vi "Image or Table Caption V2.vi"(0 "PDF Report IN":refnum<class "PDF Report Class.lvclass">, 2 "Image or Table":T1, 9 "Caption IN":string, 11 "error IN":errorcluster) -> (4 "PDF Report OUT":refnum<class "PDF Report Class.lvclass">, 6 "PdfpTable Refnum":refnum<k24>, 15 "error OUT":errorcluster)   [LabVIEW 2019, in "Exaprom PDF.lvlib"]
doc: "Version 2.0\nDeveloped by Jean-Marc Simard\nCopyright © 2012, Exaprom Inc.\nAll rights reserved.\nLicense: BSD\n\nWith iTextSharp 4.1.6 (http://itextsharp.sourceforge.net)\nunder Mozilla Public License Version 1.1\n(http://www.mozilla.org/MPL/MPL-1.1.html)"
uses:
  LV Class/PDF Report Class/PDF Report Class.lvclass
  C:/work/niobrara_lv/labview pdf writer fixing/DLL/itextsharp.dll
  DLL/itextsharp.dll
  Not  in the library/Images for controls/Image or Table.ctl
  Controls/Table Controls/Table properties.ctl
  Controls/Table Controls/Table position.ctl
  Controls/Table Controls/Cell, Alignment, LS and Font.ctl
  Controls/Table Controls/Cell Alignment 20px.ctl
  Controls/Table Controls/Text vertical arrangement.ctl
  Controls/Text Controls/Line spacing.ctl
  Controls/Table Controls/Merge Horizontal.ctl
  Controls/Font Controls/Font complete cluster.ctl
  Controls/Font Controls/Font size.ctl
  Controls/Font Controls/Font color.ctl
  Controls/Font Controls/Type and encoding.ctl
  Controls/Text Controls/Unicode/Type and run direction.ctl
  Controls/Table Controls/Cell Cluster.ctl
  Exaprom PDF.lvlib
  Controls/Table Controls/Cell Appearance.ctl
  Controls/Table Controls/Cell Border 20 px.ctl
  Controls/Table Controls/Cell Type, Alignment and LS.ctl
  Controls/Table Controls/Merge Vertical.ctl
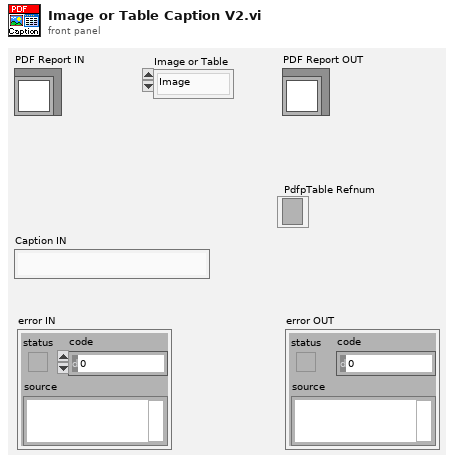
[diagram p1: front panel]
types:
  T1 = typedef "Exaprom PDF.lvlib/Image or Table.ctl" = enum16{"Image", "Table"}
  T2 = typedef "Exaprom PDF.lvlib/Cell Cluster.ctl" = cluster{"Font Ref":refnum<k24>, "Close font ref":bool, "Type and run direction":T3, "Cell Alignment":T4, "Text rotation":T5, "Leading":T6, "PdfP Cell ref":refnum<k24>, "Colspan":i8}
  T3 = typedef "Exaprom PDF.lvlib/Type and run direction.ctl" = enum16{"Select", "ASCII", "UTF-16", "UTF-16 (default)", "UTF-16 (LTR)", "UTF-16 (RTL)"}
  T4 = typedef "Exaprom PDF.lvlib/Cell Alignment 20px.ctl" = u16
  T5 = typedef "Exaprom PDF.lvlib/Text vertical arrangement.ctl" = enum16{"None", "Clockwise", "Counterclockwise"}
  T6 = typedef "Exaprom PDF.lvlib/Font size.ctl" = sgl
  T7 = cluster{"Row":cluster{"#":i16, "to #":i16}, "Cell [ ]":T2[]}
  T8 = typedef "Exaprom PDF.lvlib/Cell, Alignment, LS and Font.ctl" = cluster{"Text":T9, "Cell Appearance":T11, "HMerge":T13, "VMerge":T14, "Font":T15}
  T9 = typedef "Exaprom PDF.lvlib/Cell Type, Alignment and LS.ctl" = cluster{"Cell Alignment":T4, "Text rotation":T5, "Line spacing":T10}
  T10 = typedef "Exaprom PDF.lvlib/Line spacing.ctl" = enum16{"Select", "1.0", "1.5", "2.0"}
  T11 = typedef "Exaprom PDF.lvlib/Cell Appearance.ctl" = cluster{"Border":T12, "Thickness":sgl, "Color":u32, "BG":u32}
  T12 = typedef "Exaprom PDF.lvlib/Cell Border 20 px.ctl" = u16
  T13 = typedef "Exaprom PDF.lvlib/Merge Horizontal.ctl" = cluster{"From":i8, "to":i8}
  T14 = typedef "Exaprom PDF.lvlib/Merge Vertical.ctl" = cluster{"From":i8, "to":i8}
  T15 = typedef "Exaprom PDF.lvlib/Font complete cluster.ctl" = cluster{"Name":string, "Size":T6, "Color":T16, "Style":cluster{"Bold":bool, "Italic":bool, "Underline":bool, "Strikeout":bool}, "Type":T17}
  T16 = typedef "Exaprom PDF.lvlib/Font color.ctl" = u32
  T17 = typedef "Exaprom PDF.lvlib/Type and encoding.ctl" = cluster{"Type&direction":T3, "Embedded":bool, "Encoding":string}
  T18 = typedef "Exaprom PDF.lvlib/Table properties.ctl" = cluster{"Table position":T19, "SpacingBefore (points)":sgl, "SpacingAfter (points)":sgl}
  T19 = typedef "Exaprom PDF.lvlib/Table position.ctl" = i32
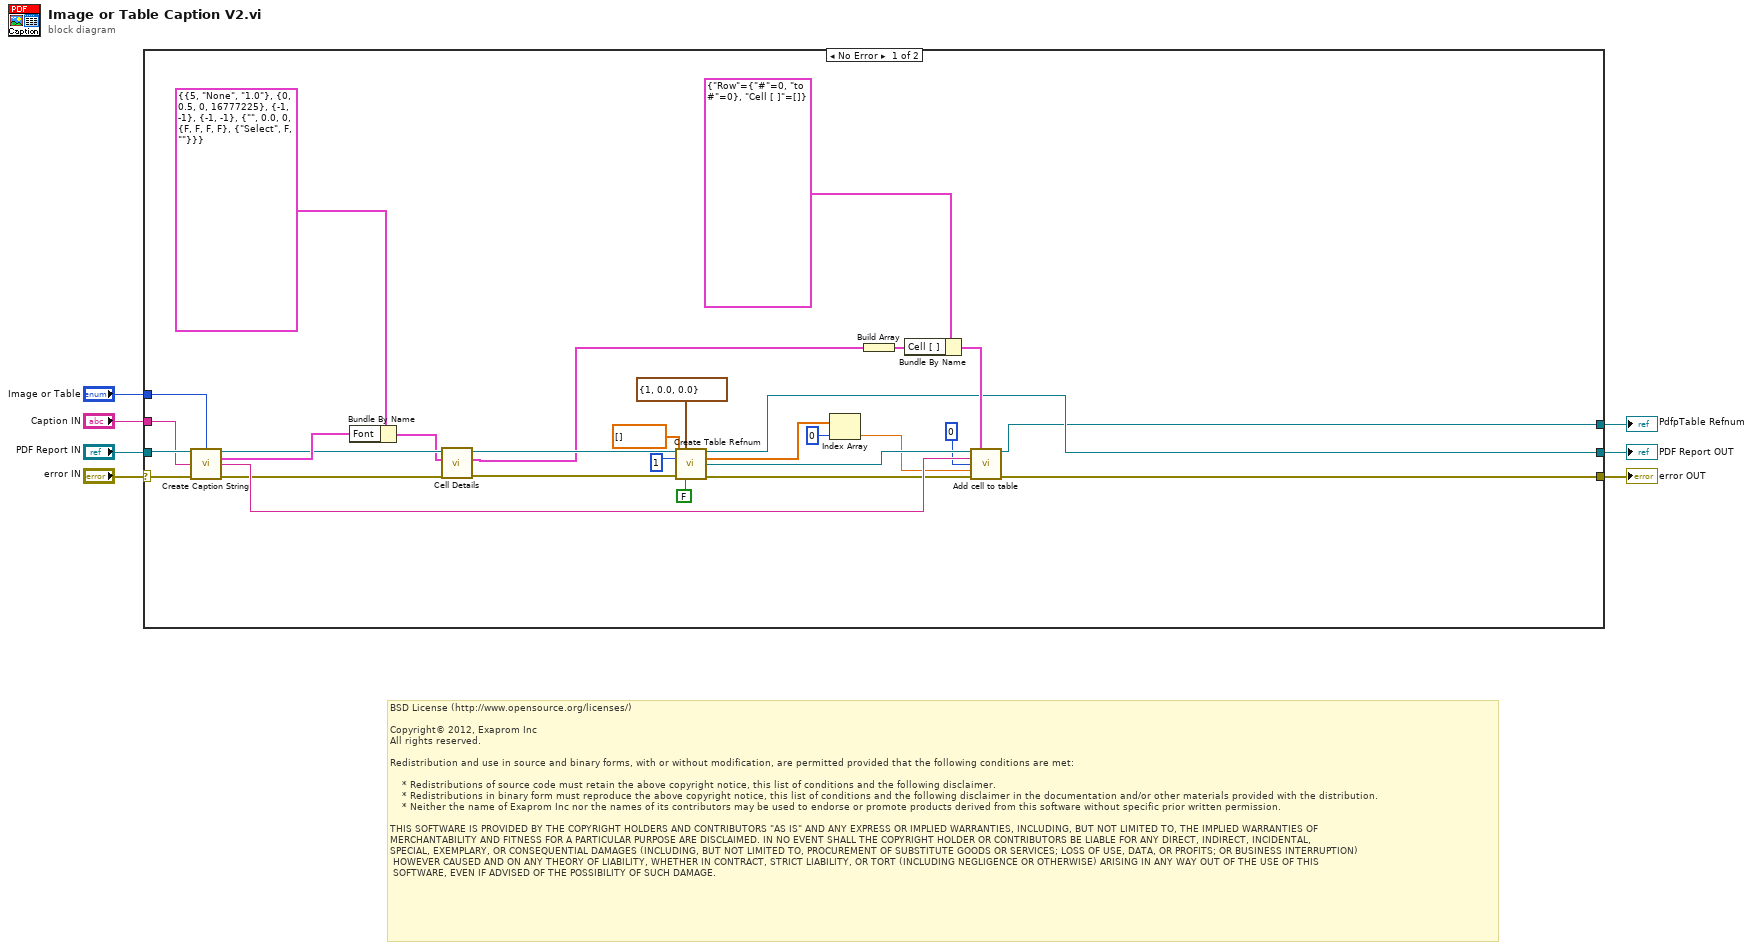
[diagram p0: block diagram]
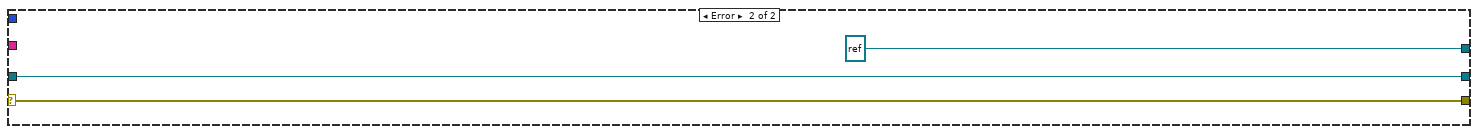
[diagram p2: hidden frame]
diagram:
  # "BSD License (http://www.opensource.org/licenses/)\n\nCopyright© 2012, Exaprom Inc\nAll rights reserved.\n\nRedistribution and use in source and binary forms, with or without modification, are permitted provided that the following conditions are met:\n\n    * Redistributions of source code must retain the above copyright notice, this list of conditions and the following disclaimer.\n    * Redistributions in binary form must reproduce the above copyright notice, this list of conditions and the following disclaimer in the documentation and/or other materials provided with the distribution.\n    * Neither the name of Exaprom Inc nor the names of its contributors may be used to endorse or promote products derived from this software without specific prior written permission.\n\nTHIS SOFTWARE IS PROVIDED BY THE COPYRIGHT HOLDERS AND CONTRIBUTORS \"AS IS\" AND ANY EXPRESS OR IMPLIED WARRANTIES, INCLUDING, BUT NOT LIMITED TO, THE IMPLIED WARRANTIES OF \nMERCHANTABILITY AND FITNESS FOR A PARTICULAR PURPOSE ARE DISCLAIMED. IN NO EVENT SHALL THE COPYRIGHT HOLDER OR CONTRIBUTORS BE LIABLE FOR ANY DIRECT, INDIRECT, INCIDENTAL,\nSPECIAL, EXEMPLARY, OR CONSEQUENTIAL DAMAGES (INCLUDING, BUT NOT LIMITED TO, PROCUREMENT OF SUBSTITUTE GOODS OR SERVICES; LOSS OF USE, DATA, OR PROFITS; OR BUSINESS INTERRUPTION)\n HOWEVER CAUSED AND ON ANY THEORY OF LIABILITY, WHETHER IN CONTRACT, STRICT LIABILITY, OR TORT (INCLUDING NEGLIGENCE OR OTHERWISE) ARISING IN ANY WAY OUT OF THE USE OF THIS\n SOFTWARE, EVEN IF ADVISED OF THE POSSIBILITY OF SUCH DAMAGE."
  n1 = case shown="No Error" "error IN" {
    selector: "error IN" -> [w36 w39]
    tunnel: [w10 w38] -> w7
    tunnel: "Caption IN" -> [w34 _]
    tunnel: "PDF Report IN" -> [w35 w38]
    tunnel: [w11 w39] -> w4
    tunnel: [w9 refnum<k24> refnum ("new reference")] -> w2
    tunnel: "Image or Table" -> [w33 _]
    frame No Error {
      n2 = call "Create Caption String.vi"("PDF Report IN"=w35, "Image or Table"=w33, "Caption IN"=w34, "error in (no error)"=w36) -> ("PDF Report OUT"=w17:refnum<class "PDF Report Class.lvclass">, "Font"=w28:T15, "Caption OUT"=w23:string, "error out"=w18:errorcluster)  [unwired: 8 in]
      n3 = Bundle By Name(cluster=T8 {"Text"={"Cell Alignment"=5, "Text rotation"=enum."None", "Line spacing"=enum."1.0"}, "Cell Appearance"={"Border"=0, "Thickness"=0.5, "Color"=0, "BG"=16777225}, "HMerge"={"From"=-1, "to"=-1}, "VMerge"={"From"=-1, "to"=-1}, "Font"={"Name"="", "Size"=0.0, "Color"=0, "Style"={"Bold"=FALSE, "Italic"=FALSE, "Underline"=FALSE, "Strikeout"=FALSE}, "Type"={"Type&direction"=enum."Select", "Embedded"=FALSE, "Encoding"=""}}} ("Cell, Alignment, LS and Font"), "Font"=w28) -> (w16:T8)
      n4 = call "Cell Details.vi"("error in (no error)"=w18, "Cell, Alignment, LS and Font"=w16, "PDF Report"=w17) -> ("error out"=w15:errorcluster, "Cell Cluster"=w13:T2, "PDF Report duplicate"=w14:refnum<class "PDF Report Class.lvclass">)  [unwired: 6 out]
      n5 = call "Create Table Refnum.vi"("PDF Report"=w14, "Table properties"=T18 {"Table position"=1, "SpacingBefore (points)"=0.0, "SpacingAfter (points)"=0.0}, "numColumns"=1, "columnWidth [ ]"=sgl[] [], "error in (no error)"=w15, "Repeat on each new page?"=FALSE) -> ("PDF Report duplicate"=w10:refnum<class "PDF Report Class.lvclass">, "columnWidth (points)"=w22:sgl[], "PdfP Table ref"=w24:refnum<k24>, "error out"=w12:errorcluster)  [unwired: 6 in]
      n6 = Index Array(array=w22, index=0) -> (element=w20:sgl)
      n7 = Build Array(w13) -> (w26:T2[])
      n8 = Bundle By Name(cluster=T7 {"Row"={"#"=0, "to #"=0}, "Cell [ ]"=[]} ("Row format with ref 2"), "Cell [ ]"=w26) -> (w25:T7)
      n9 = call "Add cell to table.vi"("PdfP Table"=w24, "Row format with ref 2"=w25, "String"=w23, "i"=0, "Column Width (points)"=w20, "error in (no error)"=w12) -> ("PdfP Table duplicate"=w9:refnum<k24>, "error out"=w11:errorcluster)  [unwired: 3 in, 5 out]
    }
    frame Error {
    }
  }
  "PDF Report OUT" <- w7
  "error OUT" <- w4
  "PdfpTable Refnum" <- w2
